vi "Teleop.vi"(10 "Match Info":T1={"Autonomous Elapsed Seconds"=0.0, "TeleOp Elapsed Seconds"=0.0, "Disabled Elapsed Seconds"=0.0, "Visited Autonomous"=FALSE, "Visited TeleOp"=FALSE, "Visited Disabled"=FALSE, "Autonomous Settings"={"Autonomous Style"=enum."Independent", "VI Refnum"=refnum}}, 11 "Call Context":T2) -> ()   [LabVIEW 2014]
doc: "This VI is called for each TeleOp packet received from the DS where the robot is not disabled. It is often used to read from the joysticks and update I/O or to update setpoints for timed control loops. It should complete and return within 20 milliseconds or it may miss DS packets."
uses:
  <vilib>/Rock Robotics/WPI/DriverStation/WPI_DriverStationDerivedRobotMode.ctl
  <vilib>/Rock Robotics/WPI/DriverStation/WPI_DriverStationMatch Info.ctl
  <vilib>/Rock Robotics/WPI/RobotDrive/WPI_RobotDriveGetSetRefNum.vi
  <vilib>/Rock Robotics/WPI/Joystick/WPI_JoystickGetSetRefNum.vi
  <vilib>/Rock Robotics/Network Tables/SD Write Boolean Array.vi
  <vilib>/Rock Robotics/Network Tables/SD Write Numeric Array.vi
  <vilib>/Rock Robotics/Network Tables/SD Read Boolean.vi
  <vilib>/Rock Robotics/Network Tables/SD Read Number.vi
panel:
  out "Sample Slider 0":dbl(slide) scale=0.0..5.0
  out "Sample Boolean 1":bool
  out "Sample Boolean 0":bool
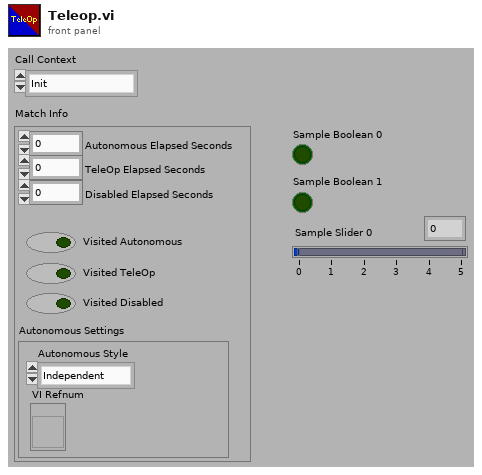
[diagram p1: front panel]
types:
  T1 = typedef "WPI_DriverStationMatch Info.ctl" = cluster{"Autonomous Elapsed Seconds":dbl, "TeleOp Elapsed Seconds":dbl, "Disabled Elapsed Seconds":dbl, "Visited Autonomous":bool, "Visited TeleOp":bool, "Visited Disabled":bool, "Autonomous Settings":cluster{"Autonomous Style":enum16{"Iterative", "Independent"}, "VI Refnum":refnum<vi>}}
  T2 = typedef "WPI_DriverStationDerivedRobotMode.ctl" = enum16{"Init", "Execute", "Stop"}
  T3 = typedef "WPI_JoystickDevRef.ctl" = cluster{"Device":T4}
  T4 = typedef "WPI_JoystickDeviceEnum.ctl" = enum16{"USB 0", "USB 1", "USB 2", "USB 3", "USB 4", "USB 5"}
  T5 = cluster{"Axes[0]":dbl, "Axes[1]":dbl, "Axes[2]":dbl, "Axes[3]":dbl, "Axes[4]":dbl, "Axes[5]":dbl, "Axes[6]":dbl, "Axes[7]":dbl, "Axes[8]":dbl}
  T6 = cluster{"Buttons[0]":bool, "Buttons[1]":bool, "Buttons[2]":bool, "Buttons[3]":bool, "Buttons[4]":bool, "Buttons[5]":bool, "Buttons[6]":bool, "Buttons[7]":bool, "Buttons[8]":bool}
  T7 = typedef "WPI_DigitalInputDevRef.ctl" = cluster{"DevStatus":errorcluster, "DIO Channel":T8, "Controller":T9}
  T8 = typedef "FPGA_DIOChannel.ctl" = enum8{"DIO 0", "DIO 1", "DIO 2", "DIO 3", "DIO 4", "DIO 5", "DIO 6", "DIO 7", "DIO 8", "DIO 9", "DIO MXP 0", "DIO MXP 1", "DIO MXP 2", "DIO MXP 3", "DIO MXP 4", "DIO MXP 5", "DIO MXP 6", "DIO MXP 7", "DIO MXP 8", "DIO MXP 9", "DIO MXP 10", "DIO MXP 11", "DIO MXP 12", "DIO MXP 13", "DIO MXP 14", "DIO MXP 15", "Invalid"}
  T9 = typedef "FPGA_TypedefDigitalModule.ctl" = enum16{"Controller 1"}
  T10 = typedef "WPI_RobotDriveDevRef.ctl" = cluster{"DevStatus":errorcluster, "Motors[]":T11[], "Square Inputs":bool, "Max Output":dbl}
  T11 = typedef "WPI_MotorControlDeviceRef.ctl" = cluster{"DeviceStatus":errorcluster, "Type":T12, "PWM":cluster{"Controller":T9, "PWM Channel":T13, "DeadBand":T14}, "CAN":cluster{"Device Number":u8, "Control Mode":T15, "Semaphore":T16, "Max Vout":dbl, "TalonSRX Control Mode":T17}, "Invert":bool, "TransformRef":T18, "InvTransformRef":T18}
  T12 = typedef "WPI_MotorControlType.ctl" = enum16{"PWM", "CAN", "CANTalonSRX"}
  T13 = typedef "FPGA_DIOPWMChannel.ctl" = enum8{"PWM 0", "PWM 1", "PWM 2", "PWM 3", "PWM 4", "PWM 5", "PWM 6", "PWM 7", "PWM 8", "PWM 9", "PWM MXP 0", "PWM MXP 1", "PWM MXP 2", "PWM MXP 3", "PWM MXP 4", "PWM MXP 5", "PWM MXP 6", "PWM MXP 7", "PWM MXP 8", "PWM MXP 9", "Invalid"}
  T14 = typedef "WPI_PWMDeadband.ctl" = cluster{"Name":string, "maxPositivePwm":i32, "minPositivePwm":i32, "centerPwm":i32, "maxNegativePwm":i32, "minNegativePwm":i32, "angularRange":u16}
  T15 = typedef "WPI_CANJaguar_ControlMode.ctl" = enum8{"Percent VBus", "Current", "Speed", "Position", "Voltage"}
  T16 = typedef "Semaphore RefNum" = refnum<k1>
  T17 = typedef "WPI_CANTalonSRX_APIControlMode.ctl" = enum8{"Percent VBus", "Speed", "Position", "Slave", "Unchanged / Invalid"}
  T18 = typedef "WPI_PWMTransform_ConPane.ctl" = refnum<vi>
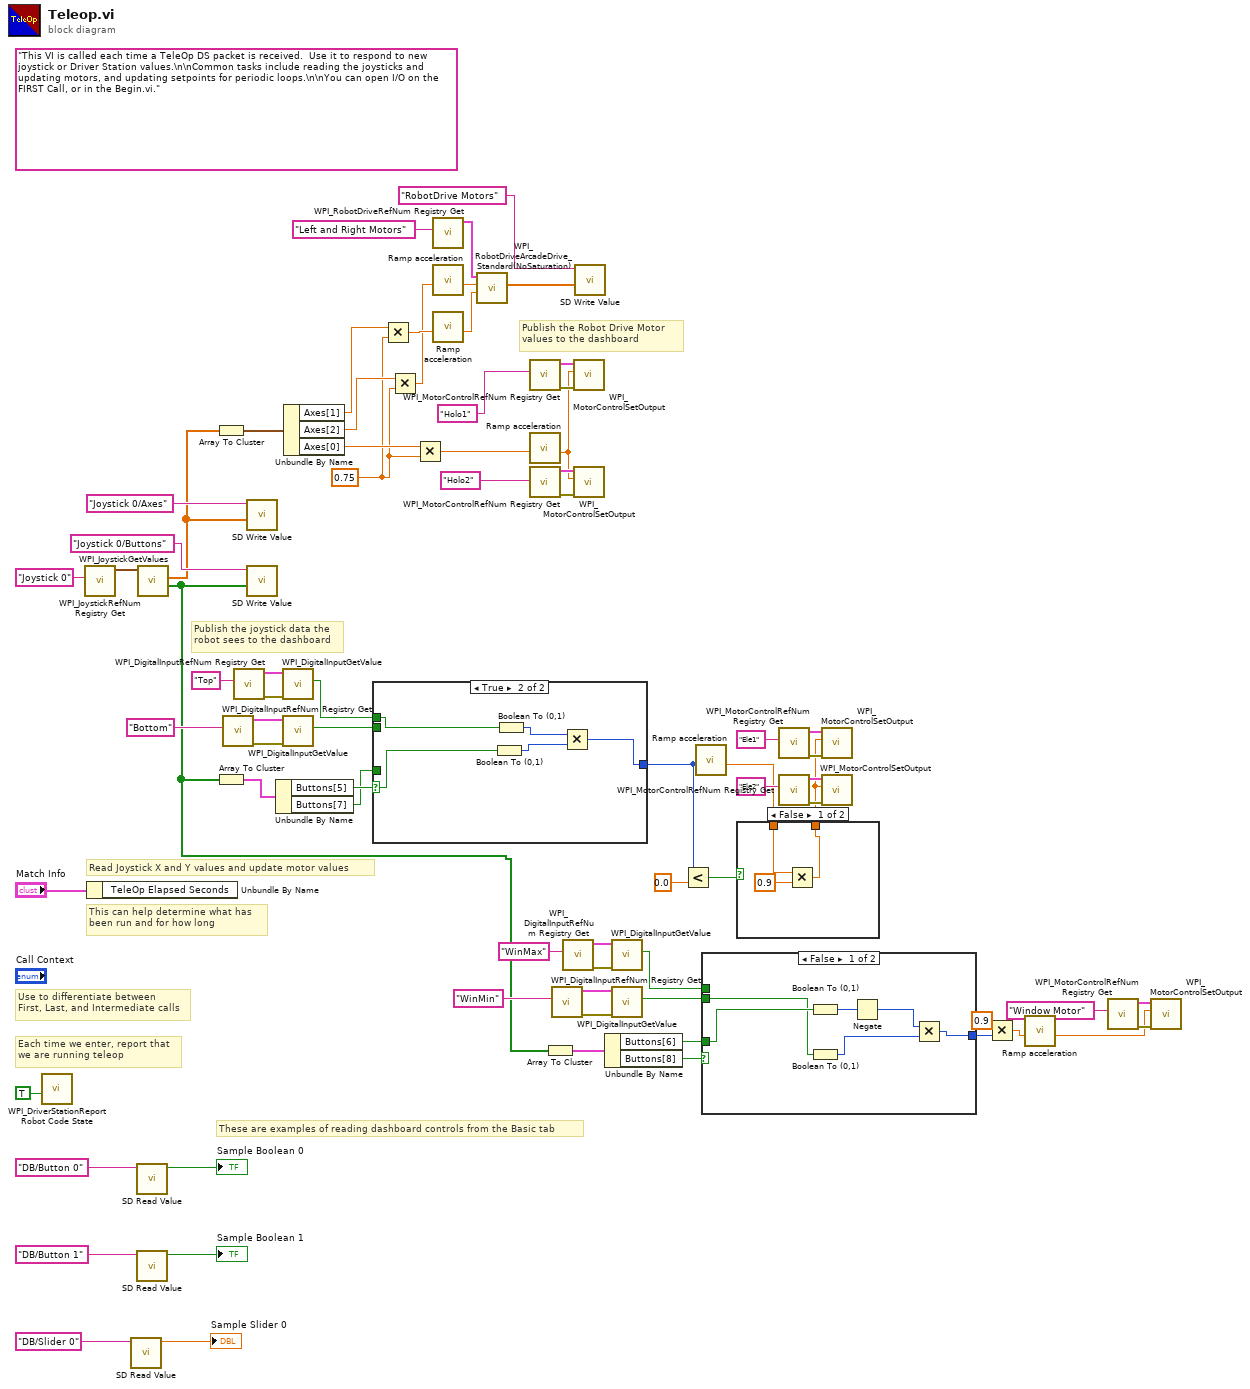
[diagram p0: block diagram]
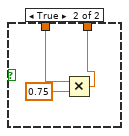
[diagram p2: hidden frame]
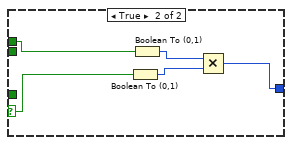
[diagram p3: hidden frame]
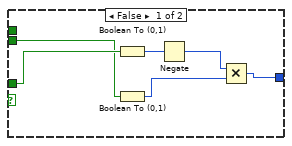
[diagram p4: hidden frame]
diagram:
  w48 = 0.75
  (unwired) "This VI is called each time a TeleOp DS packet is received.  Use it to respond to new joystick or Driver Station values.\n\nCommon tasks include reading the joysticks and updating motors, and updating setpoints for periodic loops.\n\nYou can open I/O on the FIRST Call, or in the Begin.vi."
  # "These are examples of reading dashboard controls from the Basic tab"
  # "Publish the Robot Drive Motor\nvalues to the dashboard"
  # "Publish the joystick data the\nrobot sees to the dashboard"
  # "Each time we enter, report that\nwe are running teleop"
  # "Use to differentiate between\nFirst, Last, and Intermediate calls"
  # "This can help determine what has\nbeen run and for how long"
  # "Read Joystick X and Y values and update motor values"
  n1 = call <vilib>:"WPI_DriverStationReport Robot Code State.vi"("TeleOp"=TRUE ("Autonomous")) -> ()  [unwired: 10 in, 1 out]
  n2 = call <vilib>:"WPI_JoystickRefNum Registry Get.vi"("refnum name"="Joystick 0") -> ("JoystickDevRef"=w71:T3)  [unwired: 1 in, 9 out]
  n3 = Unbundle By Name("Match Info") -> ()  [unwired: 1 out]
  n4 = call-poly <vilib>:"SD Read Value.vi"("Name"="DB/Slider 0" ("refnum name")) -> ("Numeric"=→"Sample Slider 0":dbl)  [unwired: 8 in, 2 out]
  n5 = call-poly <vilib>:"SD Read Value.vi"("Name"="DB/Button 0" ("refnum name")) -> ("Boolean"=→"Sample Boolean 0":bool)  [unwired: 8 in, 2 out]
  n6 = call-poly <vilib>:"SD Read Value.vi"("Name"="DB/Button 1" ("refnum name")) -> ("Boolean"=→"Sample Boolean 1":bool)  [unwired: 8 in, 2 out]
  n7 = call <vilib>:"WPI_JoystickGetValues.vi"("JoystickDevRef"=w71) -> ("Buttons"=w8:bool[], "Axes"=w59:dbl[])  [unwired: 6 in, 3 out]
  n8 = Array To Cluster(array=w59) -> (cluster=w58:T5)
  n9 = Array To Cluster(array=w8) -> (cluster=w26:T6)
  n10 = call <vilib>:"WPI_DigitalInputRefNum Registry Get.vi"("refnum name"="Bottom") -> ("error out"=w37:errorcluster, "DigitalInputDevRef"=w38:T7)  [unwired: 9 in]
  n11 = call <vilib>:"WPI_DigitalInputRefNum Registry Get.vi"("refnum name"="Top") -> ("error out"=w39:errorcluster, "DigitalInputDevRef"=w40:T7)  [unwired: 9 in]
  n12 = call-poly <vilib>:"SD Write Value.vi"("Numeric Array"=w59, "Name"="Joystick 0/Axes") -> ()  [unwired: 8 in, 2 out]
  n13 = call-poly <vilib>:"SD Write Value.vi"("Boolean Array"=w8, "Name"="Joystick 0/Buttons") -> ()  [unwired: 8 in, 2 out]
  n14 = Unbundle By Name(w26) -> ("Buttons[5]"=w41:bool, "Buttons[7]"=w7:bool)
  n15 = call <vilib>:"WPI_DigitalInputGetValue.vi"("error in (no error)"=w39, "DigitalInputDevRef"=w40) -> ("Value"=w27:bool)  [unwired: 7 in, 2 out]
  n16 = call <vilib>:"WPI_DigitalInputGetValue.vi"("error in (no error)"=w37, "DigitalInputDevRef"=w38) -> ("Value"=w28:bool)  [unwired: 7 in, 2 out]
  n17 = Unbundle By Name(w58) -> ("Axes[1]"=w51:dbl, "Axes[2]"=w50:dbl, "Axes[0]"=w49:dbl)
  n18 = case shown="True" w41 {
    selector: w41 -> [_ w86]
    tunnel: w7 -> [w80 _]
    tunnel: [w76 w82] -> w3
    tunnel: w28 -> [w79 _]
    tunnel: w27 -> [_ w85]
    frame False {
      n19 = Boolean To (0,1)(Boolean=w80) -> (0, 1=w81:i16)
      n20 = Boolean To (0,1)(Boolean=w79) -> (0, 1=w77:i16)
      n21 = Negate(x=w81) -> (-x=w78:i16)
      n22 = Multiply(x=w78, y=w77) -> (x*y=w76:i16)
    }
    frame True {
      n23 = Boolean To (0,1)(Boolean=w86) -> (0, 1=w83:i16)
      n24 = Boolean To (0,1)(Boolean=w85) -> (0, 1=w84:i16)
      n25 = Multiply(x=w84, y=w83) -> (x*y=w82:i16)
    }
  }
  n26 = Multiply(x=w51, y=w48) -> (x*y=w46:dbl)
  n27 = Multiply(x=w50, y=w48) -> (x*y=w45:dbl)
  n28 = Multiply(x=w49, y=w48) -> (x*y=w43:dbl)
  n29 = call <vilib>:"WPI_RobotDriveRefNum Registry Get.vi"("refnum name"="Left and Right Motors") -> ("RobotDriveDevRef"=w73:T10)  [unwired: 1 in, 9 out]
  n30 = call "Ramp acceleration.vi"("Numeric"=w45) -> ("Numeric 2"=w44:dbl)  [unwired: 10 in]
  n31 = call "Ramp acceleration.vi"("Numeric"=w46) -> ("Numeric 2"=w47:dbl)  [unwired: 10 in]
  n32 = call <vilib>:"WPI_RobotDriveArcadeDrive_Standard(NoSaturation).vi"("Y axis value"=w47, "X axis value"=w44, "RobotDriveDevRef"=w73) -> ("Motor Values"=w62:dbl[])  [unwired: 1 in, 7 out]
  n33 = call <vilib>:"WPI_MotorControlRefNum Registry Get.vi"("refnum name"="Holo1") -> ("error out"=w56:errorcluster, "MotorControlDevRef"=w57:T11)  [unwired: 9 in]
  n34 = call "Ramp acceleration.vi"("Numeric"=w43) -> ("Numeric 2"=w42:dbl)  [unwired: 10 in]
  n35 = call <vilib>:"WPI_MotorControlRefNum Registry Get.vi"("refnum name"="Holo2") -> ("error out"=w53:errorcluster, "MotorControlDevRef"=w54:T11)  [unwired: 9 in]
  n36 = Array To Cluster(array=w8) -> (cluster=w13:T6)
  n37 = call <vilib>:"WPI_DigitalInputRefNum Registry Get.vi"("refnum name"="WinMin") -> ("error out"=w21:errorcluster, "DigitalInputDevRef"=w22:T7)  [unwired: 9 in]
  n38 = call <vilib>:"WPI_DigitalInputRefNum Registry Get.vi"("refnum name"="WinMax") -> ("error out"=w23:errorcluster, "DigitalInputDevRef"=w24:T7)  [unwired: 9 in]
  n39 = call <vilib>:"WPI_MotorControlSetOutput.vi"("error in (no error)"=w56, "Output"=w42, "MotorControlDevRef"=w57) -> ()  [unwired: 6 in, 3 out]
  n40 = call <vilib>:"WPI_MotorControlSetOutput.vi"("error in (no error)"=w53, "Output"=w42, "MotorControlDevRef"=w54) -> ()  [unwired: 6 in, 3 out]
  n41 = call-poly <vilib>:"SD Write Value.vi"("Numeric Array"=w62, "Name"="RobotDrive Motors") -> ()  [unwired: 8 in, 2 out]
  n42 = Unbundle By Name(w13) -> ("Buttons[6]"=w25:bool, "Buttons[8]"=w6:bool)
  n43 = call <vilib>:"WPI_DigitalInputGetValue.vi"("error in (no error)"=w23, "DigitalInputDevRef"=w24) -> ("Value"=w14:bool)  [unwired: 7 in, 2 out]
  n44 = call <vilib>:"WPI_DigitalInputGetValue.vi"("error in (no error)"=w21, "DigitalInputDevRef"=w22) -> ("Value"=w15:bool)  [unwired: 7 in, 2 out]
  n45 = Less?(x=w3, y=0.0) -> (x < y?=w5:bool)
  n46 = call "Ramp acceleration.vi"("Numeric"=w3) -> ("Numeric 2"=w1:dbl)  [unwired: 10 in]
  n47 = case shown="False" w6 {
    selector: w6 -> [_ w97]
    tunnel: w25 -> [w91 _]
    tunnel: [w87 w93] -> w11
    tunnel: w15 -> [w90 _]
    tunnel: w14 -> [_ w96]
    frame False {
      n48 = Boolean To (0,1)(Boolean=w91) -> (0, 1=w92:i16)
      n49 = Boolean To (0,1)(Boolean=w90) -> (0, 1=w88:i16)
      n50 = Negate(x=w92) -> (-x=w89:i16)
      n51 = Multiply(x=w89, y=w88) -> (x*y=w87:i16)
    }
    frame True {
      n52 = Boolean To (0,1)(Boolean=w97) -> (0, 1=w94:i16)
      n53 = Boolean To (0,1)(Boolean=w96) -> (0, 1=w95:i16)
      n54 = Multiply(x=w95, y=w94) -> (x*y=w93:i16)
    }
  }
  n55 = case shown="False" w5 {
    tunnel: [w99 w103] -> w2
    tunnel: w1 -> [w100 w102]
    frame False {
      n56 = Multiply(x=w100, y=0.9) -> (x*y=w99:dbl)
    }
    frame True {
      n57 = Multiply(x=w102, y=0.75) -> (x*y=w103:dbl)
    }
  }
  n58 = call <vilib>:"WPI_MotorControlRefNum Registry Get.vi"("refnum name"="Ele1") -> ("error out"=w30:errorcluster, "MotorControlDevRef"=w31:T11)  [unwired: 9 in]
  n59 = call <vilib>:"WPI_MotorControlRefNum Registry Get.vi"("refnum name"="Ele2") -> ("error out"=w29:errorcluster, "MotorControlDevRef"=w32:T11)  [unwired: 9 in]
  n60 = call <vilib>:"WPI_MotorControlSetOutput.vi"("error in (no error)"=w30, "Output"=w2, "MotorControlDevRef"=w31) -> ()  [unwired: 6 in, 3 out]
  n61 = call <vilib>:"WPI_MotorControlSetOutput.vi"("error in (no error)"=w29, "Output"=w2, "MotorControlDevRef"=w32) -> ()  [unwired: 6 in, 3 out]
  n62 = Multiply(x=0.9, y=w11) -> (x*y=w10:dbl)
  n63 = call "Ramp acceleration.vi"("Numeric"=w10) -> ("Numeric 2"=w12:dbl)  [unwired: 10 in]
  n64 = call <vilib>:"WPI_MotorControlRefNum Registry Get.vi"("refnum name"="Window Motor") -> ("error out"=w16:errorcluster, "MotorControlDevRef"=w17:T11)  [unwired: 9 in]
  n65 = call <vilib>:"WPI_MotorControlSetOutput.vi"("error in (no error)"=w16, "Output"=w12, "MotorControlDevRef"=w17) -> ()  [unwired: 6 in, 3 out]
